vi "WaitMessage.vi"(11 "stop":bool) -> (0 "error in (no error) 2":errorcluster)   [LabVIEW 2022 SP3]
panel:
  # "Please wait while the system aligns itself"
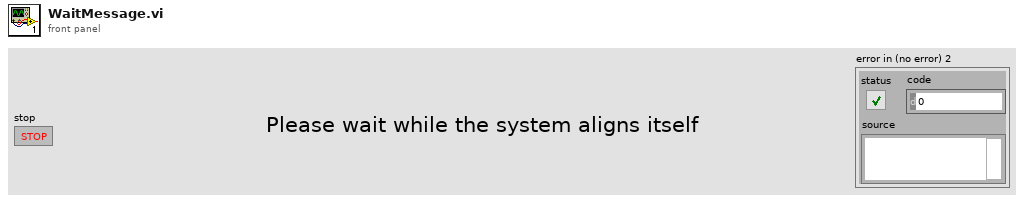
[diagram p1: front panel]
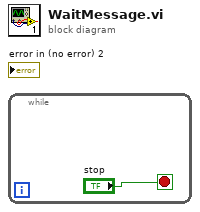
[diagram p0: block diagram]
diagram:
  n1 = while {
    stop <- "stop" stop-if-true
  }
